vi "Scope Config ReadDC.vi"(8 "error in (no error)":errorcluster, 11 "Actor_Scope in":refnum<class "Actor_Scope.lvclass">) -> (0 "error out":errorcluster, 3 "Actor_Scope out":refnum<class "Actor_Scope.lvclass">)   [LabVIEW 2020, in "Actor_Scope.lvlib" / "Actor_Scope.lvclass"]
uses:
  Actor_Scope.lvclass
  C:/Program Files/National Instruments/LabVIEW 2020/vi.lib/ActorFramework/Actor/Actor.lvclass
  Scope_Event.ctl
  Actor_Scope.lvclass/Actor_Scope.ctl
  <vilib>/ActorFramework/Actor/Actor.lvclass/Actor.ctl
  <instrlib>/Agilent 8000 Series/Agilent 8000 Series.lvlib
  <vilib>/ActorFramework/Actor/Actor.lvclass
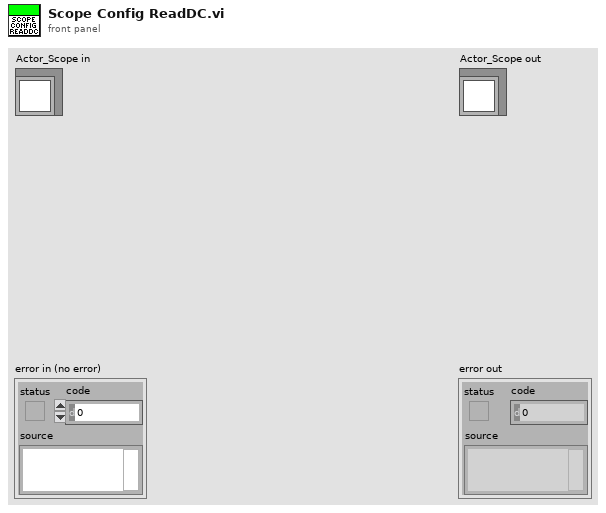
[diagram p1: front panel]
types:
  T1 = typedef "Actor_Scope.lvlib/Actor_Scope.lvclass/Scope_Event.ctl" = enum16{"General Event", "Inited", "Error", "Wfm Acq Complete"}
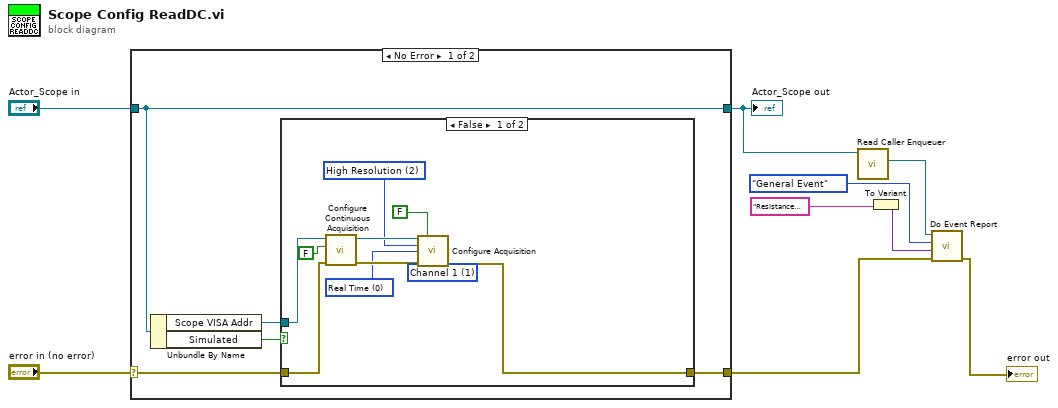
[diagram p0: block diagram]
diagram:
  n1 = case shown="No Error" "error in (no error)" {
    selector: "error in (no error)" -> [w12 w26]
    tunnel: [w11 w26] -> w2
    tunnel: [w14 w25] -> w3
    tunnel: "Actor_Scope in" -> [w14 w25]
    frame No Error {
      n2 = Unbundle By Name(w14) -> ("Scope VISA Addr"=w10:refnum<visa-resource-name>, "Simulated"=w13:bool)
      n3 = case shown="False" w13 {
        tunnel: w12 -> [w21 w24]
        tunnel: [w15 w24] -> w11
        tunnel: w10 -> [w22 _]
        frame False {
          (unwired) 1 items=["Channel 1"=1, "Channel 2"=2, "Channel 3"=3, "Channel 4"=4, "Digital 0"=13, "Digital 1"=14, "Digital 2"=15, "Digital 3"=16, "Digital 4"=17, "Digital 5"=18, "Digital 6"=19, "Digital 7"=20, "Digital 8"=21, "Digital 9"=22, "Digital 10"=23, "Digital 11"=24, "Digital 12"=25, "Digital 13"=26, "Digital 14"=27, "Digital 15"=28, "Aux"=29, "Line"=30] ("Trigger Source (1: Channel 1)")
          w17 = u16 0 items=["Real Time", "Equivalent Time", "Segment"] ("Sampling Mode  (0: Real Time)")
          w18 = u16 2 items=["Normal", "Peak Detect", "High Resolution"] ("Acquisition Type (0: Normal)")
          n4 = call <instrlib>:"Configure Continuous Acquisition.vi"("error in (no error)"=w21, "Enable Continuous Acquisition Mode (T:Enable)"=FALSE, "VISA resource name"=w22) -> ("error out"=w19:errorcluster, "VISA resource name out"=w20:refnum<visa-resource-name>)  [unwired: 7 in]
          n5 = call <instrlib>:"Configure Acquisition.vi"("VISA resource name"=w20, "Enable Analog Averaging (Disable)"=FALSE, "Acquisition Type (0: Normal)"=w18, "Sampling Mode  (0: Real Time)"=w17, "error in (no error)"=w19) -> ("error out"=w15:errorcluster)  [unwired: 9 in, 1 out]
        }
        frame True {
        }
      }
    }
    frame Error {
    }
  }
  "Actor_Scope out" <- w3
  n6 = call <vilib>:"Read Caller Enqueuer.vi"("Actor"=w3) -> ("Caller Enqueuer"=w6:refnum<class "Message Enqueuer.lvclass">)  [unwired: 10 in]
  n7 = To Variant(anything="Resistance Meas Configured") -> (Variant=w4:variant)
  n8 = call "Do Event Report.vi"("error in (no error)"=w2, "Event Data"=w4, "Scope Events"=Scope_Event."General Event", "Caller Enqueuer"=w6) -> ("error out"=→"error out":errorcluster)  [unwired: 6 in, 1 out]
